vi "Matrix Inverse v1.2.vi"() -> ()   [LabVIEW 2020]
uses:
  <vilib>/Analysis/Matrix/Datatypes/RealMatrix.ctl
  <vilib>/Analysis/baseanly.llb/Mean (DBL).vi
  <vilib>/Analysis/Matrix/Numeric/Conversions/Array To Matrix - RA2.vi
  <vilib>/Analysis/baseanly.llb/Real Inverse Matrix.vi
  <vilib>/Analysis/Matrix/Numeric/Conversions/Matrix To Array - RM.vi
  <vilib>/Analysis/NI_AALBase.lvlib
  <vilib>/Analysis/Matrix/NI_Matrix.lvlib
panel:
  out "pt - pt error":sgl[][](array[numeric])
  out "percent error":dbl format="%0.2f"
  out "x > y?":bool
  out "divide by zero detected":bool
  out "Joint Matrix":sgl[][](array[numeric])
  out "A":T1
  out "sum of error":sgl
  out "inv(A) LABVIEW-FPGA":sgl[][](array[numeric])
  out "inv(A) LABVIEW":T1
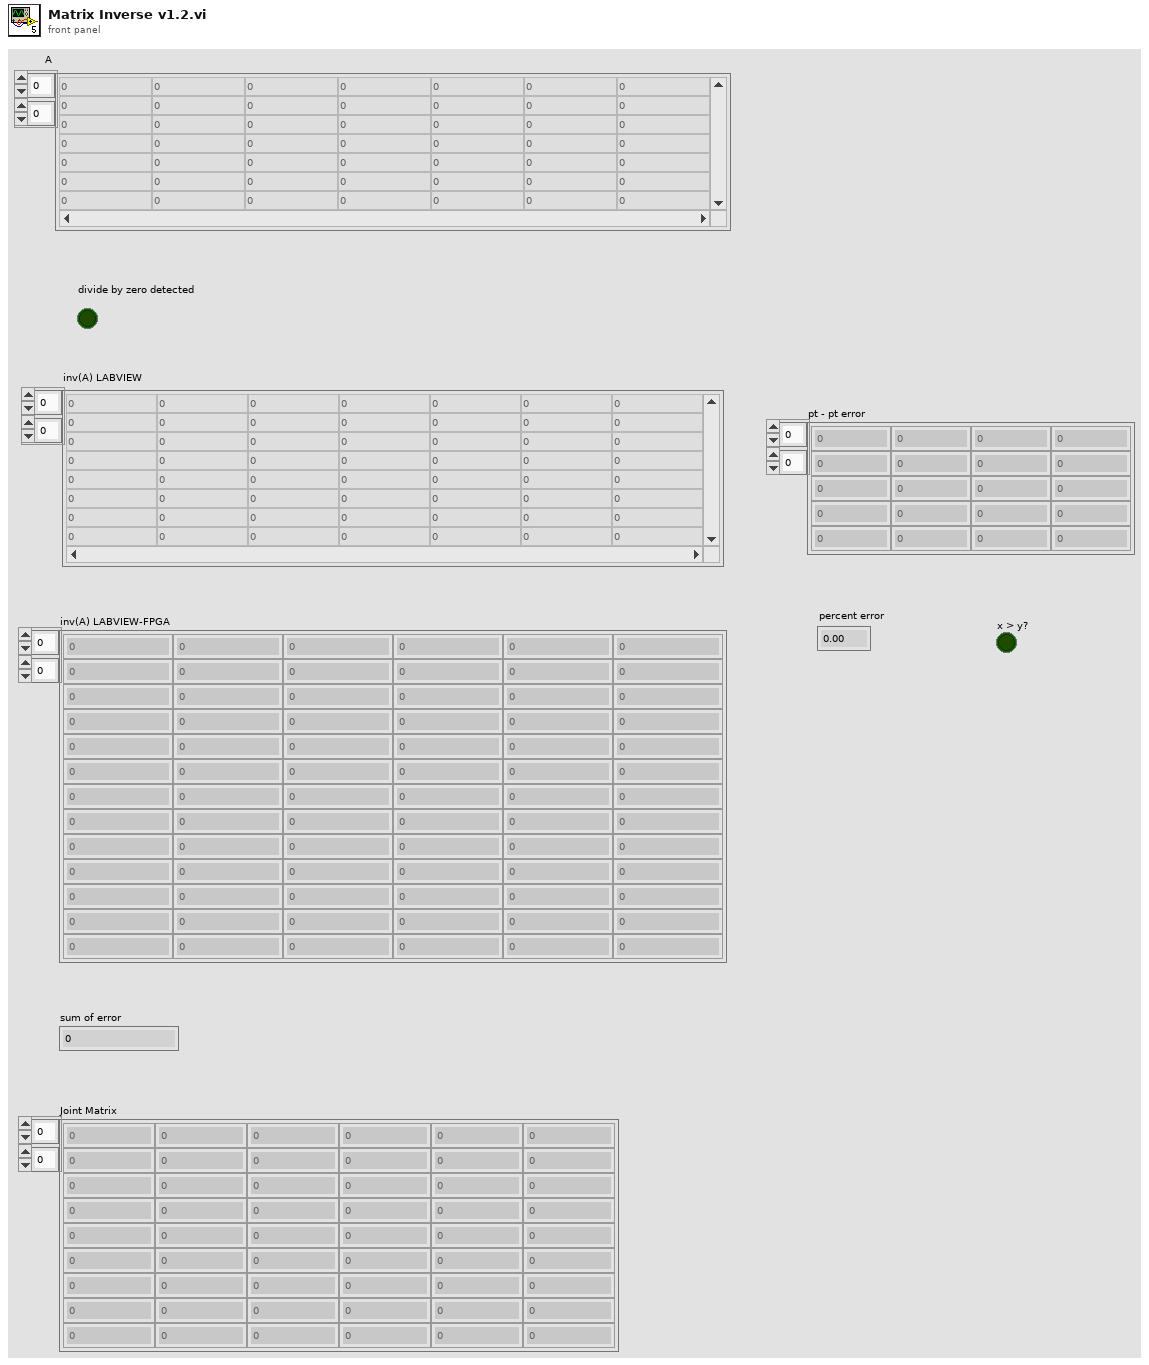
[diagram p1: front panel]
types:
  T1 = typedef "NI_Matrix.lvlib/RealMatrix.ctl" = dbl[][]
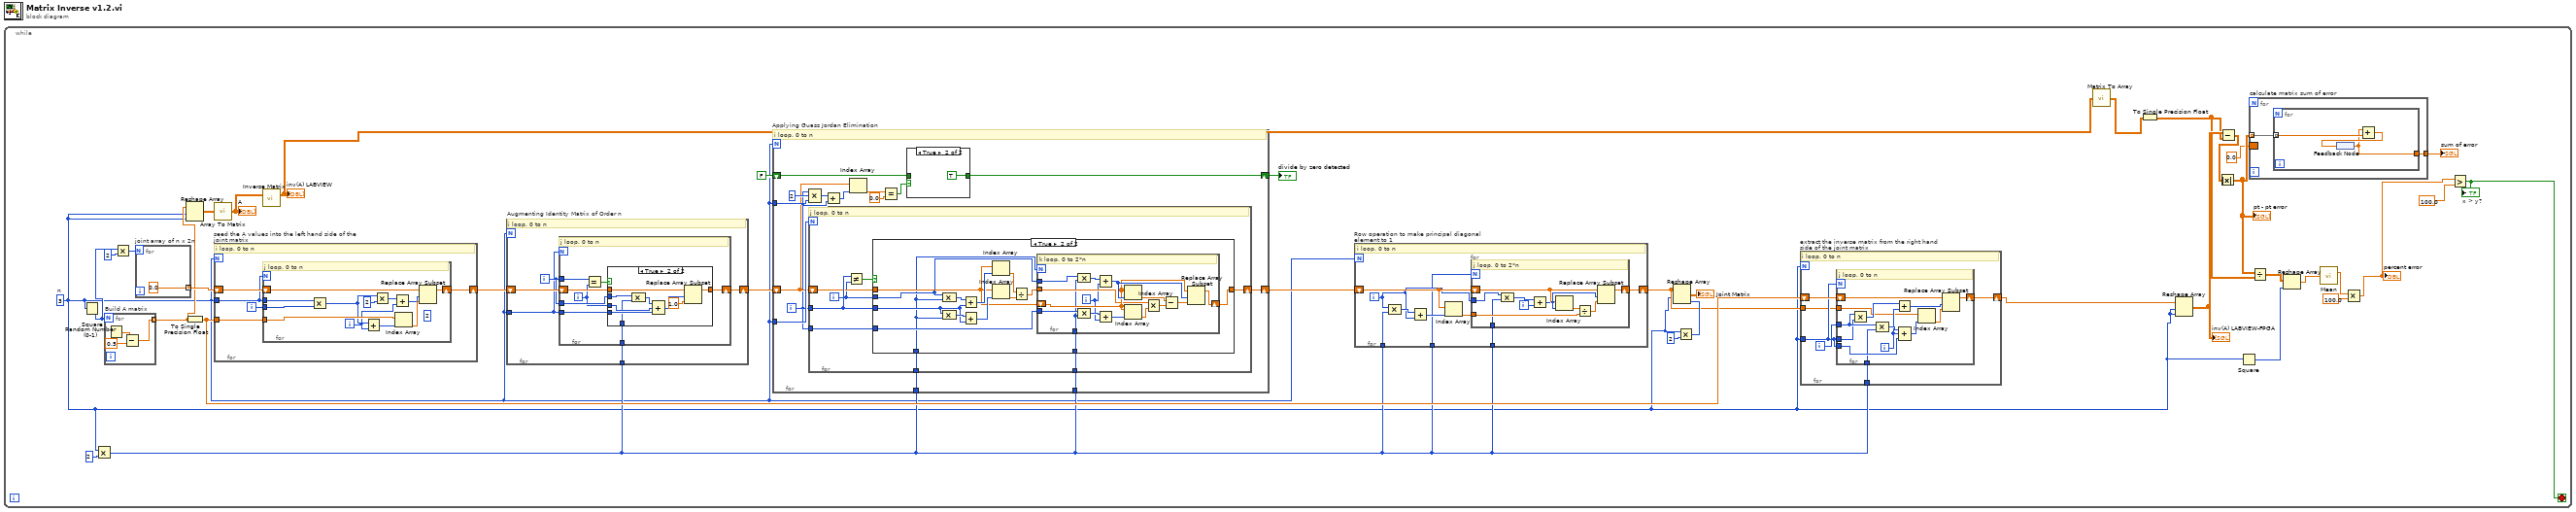
[diagram p0: block diagram]
diagram:
  n1 = while {
    stop <- w12 stop-if-true
    w4 = 3  # n
    n2 = Square(x=w4) -> (x^2=w17:i32)
    n3 = Multiply(x=w4, y=2) -> (x*y=w15:i32)
    n4 = for "Build A matrix" {
      N: w17 -> [_]
      tunnel: [w172] -> w24 mode=indexing
      n5 = Random Number (0-1)() -> (number: 0 to 1=w174:dbl)
      n6 = Subtract(x=w174, y=0.5) -> (x-y=w172:dbl)
    }
    n7 = Multiply(x=w17, y=2) -> (x*y=w31:i32)
    n8 = for "joint array of n x 2n" {
      N: w31 -> [_]
      tunnel: [sgl 0.0] -> w30 mode=indexing
    }
    n9 = Reshape Array(w24, w4, w4) -> (w37:dbl[][])
    n10 = To Single Precision Float(number=w24) -> (single precision float=w23:sgl[])
    n11 = call-poly <vilib>:"Array To Matrix.vi"("Real 2D Array"=w37) -> ("Real Matrix"=w36:T1)
    "A" <- w36
    n12 = for "seed the A values into the left hand side of the joint matrix" {
      N: w4 -> [_]
      shift-right: [w134] -> w29
      shift-left: w30 -> [w135]
      tunnel: w4 -> [w133]
      tunnel: w23 -> [w132]
      i -> [w131]
      # "i loop, 0 to n"
      n13 = for {
        N: w133 -> [_]
        shift-right: [w146] -> w134
        shift-left: w135 -> [w147]
        tunnel: w133 -> [w143]
        tunnel: w132 -> [w145]
        tunnel: w131 -> [w144]
        i -> [w137]
        (unwired) 2
        # "j loop, 0 to n"
        n14 = Multiply(x=w143, y=w144) -> (x*y=w139:i32)
        n15 = Add(x=w139, y=w137) -> (x+y=w142:i32)
        n16 = Multiply(x=w139, y=2) -> (x*y=w138:i32)
        n17 = Add(x=w138, y=w137) -> (x+y=w136:i32)
        n18 = Index Array(array=w145, index=w142) -> (element=w141:sgl)
        n19 = Replace Array Subset(array=w147, new element=w141, index=w136) -> (w146:sgl[])
      }
    }
    n20 = call-poly <vilib>:"Inverse Matrix.vi"("Input Matrix"=w36) -> ("Inverse Matrix"=w19:T1)  [unwired: 1 in, 1 out]
    "inv(A) LABVIEW" <- w19
    n21 = for "Augmenting Identity Matrix of Order n" {
      N: w4 -> [_]
      shift-right: [w152] -> w26
      shift-left: w29 -> [w153]
      tunnel: w4 -> [w150]
      tunnel: w15 -> [w149]
      i -> [w151]
      # "i loop, 0 to n"
      n22 = for {
        N: w150 -> [_]
        tunnel: w151 -> [w161]
        shift-right: [w158] -> w152
        shift-left: w153 -> [w159]
        tunnel: w151 -> [w157]
        tunnel: w150 -> [w156]
        tunnel: w149 -> [w154]
        i -> [w155]
        # "j loop, 0 to n"
        n23 = Equal?(x=w161, y=w155) -> (x = y?=w160:bool)
        n24 = case shown="True" w160 {
          tunnel: w159 -> [w162 w171]
          tunnel: [w162 w168] -> w158
          tunnel: w157 -> [_ w169]
          tunnel: w156 -> [_ w165]
          tunnel: w155 -> [_ w166]
          tunnel: w154 -> [_ w163]
          frame False {
          }
          frame True {
            n25 = Compound Arithmetic op=MULTIPLY(w169, w163) -> (w167:i32)
            n26 = Compound Arithmetic op=ADD(w167, w166, w165) -> (w164:i32)
            n27 = Replace Array Subset(array=w171, new element=sgl 1.0 ("new element/subarray"), index=w164) -> (w168:sgl[])
          }
        }
      }
    }
    n28 = for "Applying Guass Jordan Elimination" {
      N: w4 -> [_]
      tunnel: w4 -> [w88]
      shift-right: [w82] -> w27
      shift-left: FALSE -> [w83]
      tunnel: w4 -> [w81]
      shift-right: [w78] -> w25
      shift-left: w26 -> [w80]
      tunnel: w15 -> [w77]
      tunnel: w15 -> [w76]
      i -> [w79]
      # "i loop, 0 to n"
      n29 = Compound Arithmetic op=MULTIPLY(w79, 2 ("value"), w88) -> (w87:i32)
      n30 = for {
        N: w81 -> [_]
        tunnel: w79 -> [w98]
        tunnel: w79 -> [w94]
        shift-right: [w93] -> w78
        shift-left: w80 -> [w97]
        tunnel: w77 -> [w92]
        tunnel: w76 -> [w91]
        i -> [w95]
        # "j loop, 0 to n"
        n31 = Not Equal?(x=w98, y=w95) -> (x != y?=w96:bool)
        n32 = case shown="True" w96 {
          tunnel: w98 -> [_ w107]
          tunnel: w97 -> [w99 w106]
          tunnel: w95 -> [_ w105]
          tunnel: w94 -> [_ w103]
          tunnel: [w99 w102] -> w93
          tunnel: w92 -> [_ w101]
          tunnel: w91 -> [_ w100]
          frame False {
          }
          frame True {
            n33 = Compound Arithmetic op=MULTIPLY(w105, w101) -> (w113:i32)
            n34 = Compound Arithmetic op=MULTIPLY(w107, w101) -> (w109:i32)
            n35 = Add(x=w113, y=w107) -> (x+y=w112:i32)
            n36 = Add(x=w109, y=w107) -> (x+y=w108:i32)
            n37 = Index Array(array=w106, index=w112) -> (element=w111:sgl)
            n38 = Index Array(array=w106, index=w108) -> (element=w110:sgl)
            n39 = Divide(x=w111, y=w110) -> (x/y=w104:sgl)
            n40 = for {
              N: w101 -> [_]
              tunnel: w105 -> [w127]
              tunnel: w104 -> [w123]
              tunnel: w103 -> [w120]
              shift-right: [w115] -> w102
              shift-left: w106 -> [w125]
              tunnel: w100 -> [w114]
              i -> [w121]
              # "k loop, 0 to 2*n"
              n41 = Compound Arithmetic op=MULTIPLY(w127, w114) -> (w128:i32)
              n42 = Compound Arithmetic op=MULTIPLY(w120, w114) -> (w122:i32)
              n43 = Add(x=w128, y=w121) -> (x+y=w126:i32)
              n44 = Add(x=w122, y=w121) -> (x+y=w119:i32)
              n45 = Index Array(array=w125, index=w126) -> (element=w117:sgl)
              n46 = Index Array(array=w125, index=w119) -> (element=w124:sgl)
              n47 = Multiply(x=w123, y=w124) -> (x*y=w118:sgl)
              n48 = Subtract(x=w117, y=w118) -> (x-y=w116:sgl)
              n49 = Replace Array Subset(array=w125, new element=w116, index=w126) -> (w115:sgl[])
            }
          }
        }
      }
      n50 = Add(x=w87, y=w79) -> (x+y=w86:i32)
      n51 = Index Array(array=w80, index=w86) -> (element=w85:sgl)
      n52 = Equal?(x=w85, y=sgl 0.0) -> (x = y?=w84:bool)
      n53 = case shown="True" w84 {
        tunnel: w83 -> [w129 _]
        tunnel: [w129 TRUE] -> w82
        frame False {
        }
        frame True {
        }
      }
    }
    "divide by zero detected" <- w27
    n54 = for "Row operation to make principal diagonal element to 1" {
      N: w4 -> [_]
      shift-right: [w60] -> w21
      shift-left: w25 -> [w63]
      tunnel: w15 -> [w59]
      tunnel: w15 -> [w58]
      tunnel: w15 -> [w57]
      i -> [w62]
      # "i loop, 0 to n"
      n55 = Compound Arithmetic op=MULTIPLY(w62, w58) -> (w65:i32)
      n56 = Add(x=w65, y=w62) -> (x+y=w64:i32)
      n57 = Index Array(array=w63, index=w64) -> (element=w61:sgl)
      n58 = for {
        N: w59 -> [_]
        tunnel: w62 -> [w75]
        tunnel: w61 -> [w71]
        shift-right: [w69] -> w60
        shift-left: w63 -> [w70]
        tunnel: w57 -> [w66]
        i -> [w73]
        # "j loop, 0 to 2*n"
        n59 = Compound Arithmetic op=MULTIPLY(w75, w66) -> (w74:i32)
        n60 = Add(x=w74, y=w73) -> (x+y=w68:i32)
        n61 = Index Array(array=w70, index=w68) -> (element=w72:sgl)
        n62 = Divide(x=w72, y=w71) -> (x/y=w67:sgl)
        n63 = Replace Array Subset(array=w70, new element=w67, index=w68) -> (w69:sgl[])
      }
    }
    n64 = Multiply(x=w4, y=2) -> (x*y=w34:i32)
    n65 = Reshape Array(w21, w4, w34) -> (→"Joint Matrix":sgl[][])
    n66 = for "extract the inverse matrix from the right hand side of the joint matrix" {
      N: w4 -> [_]
      tunnel: w4 -> [w40]
      shift-right: [w42] -> w22
      shift-left: w23 -> [w43]
      tunnel: w21 -> [w39]
      tunnel: w15 -> [w38]
      i -> [w41]
      # "i loop, 0 to n"
      n67 = for {
        N: w40 -> [_]
        shift-right: [w55] -> w42
        shift-left: w43 -> [w56]
        tunnel: w41 -> [w52]
        tunnel: w40 -> [w51]
        tunnel: w40 -> [w48]
        tunnel: w39 -> [w46]
        tunnel: w38 -> [w44]
        i -> [w49]
        # "j loop, 0 to n"
        n68 = Multiply(x=w52, y=w51) -> (x*y=w54:i32)
        n69 = Compound Arithmetic op=MULTIPLY(w52, w44) -> (w50:i32)
        n70 = Add(x=w54, y=w49) -> (x+y=w53:i32)
        n71 = Compound Arithmetic op=ADD(w50, w49, w48) -> (w47:i32)
        n72 = Index Array(array=w46, index=w47) -> (element=w45:sgl)
        n73 = Replace Array Subset(array=w56, new element=w45, index=w53) -> (w55:sgl[])
      }
    }
    n74 = call-poly <vilib>:"Matrix To Array.vi"("Real Matrix"=w19) -> ("Real 2D Array"=w18:dbl[][])
    n75 = To Single Precision Float(number=w18) -> (single precision float=w9:sgl[][])
    n76 = Reshape Array(w22, w4, w4) -> (w11:sgl[][])
    "inv(A) LABVIEW-FPGA" <- w11
    n77 = Subtract ("Subtract.vi")(x=w11, y=w9) -> (x-y=w20:sgl[][])
    n78 = Absolute Value ("Absolute Value.vi")(x=w20) -> (abs(x)=w10:sgl[][])
    "pt - pt error" <- w10
    n79 = Square(x=w4) -> (x^2=w3:i32)
    n80 = for "calculate matrix sum of error" {
      tunnel: w10 -> [w176] mode=indexing
      tunnel: [w175] -> w14
      border: sgl 0.0 -> [_]
      n81 = for {
        tunnel: w176 -> [w179] mode=indexing
        tunnel: [w177] -> w175
        n82 = feedback #1() -> (w177:sgl)
        n83 = Add(x=w177, y=w179) -> (x+y=w178:sgl)
        n84 = feedback-in #1(w178) -> ()
      }
    }
    "sum of error" <- w14
    n85 = Divide(x=w10, y=w9) -> (x/y=w8:sgl[][])
    n86 = Reshape Array(w8, w3) -> (w7:sgl[])
    n87 = call-poly <vilib>:"Mean.vi"("X"=w7) -> ("mean"=w6:dbl)  [unwired: 1 out]
    n88 = Multiply(x=w6, y=100.0) -> (x*y=w2:dbl)
    "percent error" <- w2
    n89 = Greater?(x=w2, y=sgl 100.0) -> (0:w12:bool)
    "x > y?" <- w12
  }
